vi "Lockin-4461_Multiple Inputs and Outputs_KH_functional_global_waveform_generalized_f.vi"(8 "stop":bool) -> ()   [LabVIEW 2013]
uses:
  <vilib>/Analysis/baseanly.llb/Mean (DBL).vi
  <vilib>/Analysis/2dsp.llb/Decimate (single shot).vi
  <vilib>/Analysis/2dsp.llb/Decimate (single shot, DBL).vi
  DAQ-Lockin-SubVI/Lock-in Globles Multiple Inputs and Outputs used with FGV.vi
  <vilib>/Utility/error.llb/Error Cluster From Error Code.vi
  <vilib>/measure/madcrms.llb/Basic Averaged DC-RMS for 1 Chan.vi
  <vilib>/DAQmx/write.llb/DAQmx Write (Analog 1D Wfm NChan NSamp).vi
  <vilib>/Analysis/NI_AALBase.lvlib
  <vilib>/measure/NI_MAPro.lvlib
  <userlib>/_OpenG.lib/comparison/comparison.llb/Variant Changed__ogtk.vi
panel:
  in  "Boolean":bool
  in  "`":i8(slide) scale=1.0..8.0
  in  "AI Buffer Size":dbl
  in  "order":dbl
  in  "AI Block Size":dbl
  in  "TC (s)":dbl
  in  "Cluster 2":T1
  in  "Enum":enum16{"X and Y", "R and Theta"}(ring)
  in  "Tab Control 3":enum32{"Page 1", "Page 2"}(tab)
  in  "auto controI block size":bool
  in  "zero offset":bool
  in  "measure offset":bool
  in  "reset signal?":bool
  in  "demod = AO?":bool
  in  "all frequencies same?":bool
  in  "simulate?":bool
  in  "Input Signals":i16(slide)=1 scale=1.0..20.0
  out "phase log":dbl[](array[numeric])
  in  "Tab Control 2":T2(tab)=enum."Lock-in Settings"
  in  "AI Configuration":T3(array[cluster])=[{"AI.Coupling"=10050, "AI.Max"=10.0, "AI.Min"=-10.0, "Input physical channels"="PXI1Slot2/ai0:1"}, {"AI.Coupling"=10050, "AI.Max"=10.0, "AI.Min"=-10.0, "Input physical channels"="PXI1Slot3/ai0:1"}, {"AI.Coupling"=10050, "AI.Max"=10.0, "AI.Min"=-10.0, "Input physical channels"="PXI1Slot5/ai0:1"}, {"AI.Coupling"=10050, "AI.Max"=10.0, "AI.Min"=-10.0, "Input physical channels"="PXI1Slot6/ai0:1"}] {"AI.Coupling" items=["AC"=10045, "DC"=10050, "GND"=10066]}
  in  "AO Configuration":T4(array[cluster])=[{"Output physical channels"="PXI1Slot2/ao0:1", "AO. Max"=0.1, "AO.Min"=-0.1}, {"Output physical channels"="PXI1Slot3/ao0:1", "AO. Max"=0.25, "AO.Min"=-0.25}, {"Output physical channels"="PXI1Slot5/ao0:1", "AO. Max"=0.1, "AO.Min"=-0.1}, {"Output physical channels"="PXI1Slot6/ao0:1", "AO. Max"=0.1, "AO.Min"=-0.1}]
  in  "Lockin":T5={"REF f (Hz)"=[13.0, 13.0, 13.0, 13.0, 13.0, 13.0, 13.0, 13.0], "REF phi (deg)"=[0.0, 0.0, 0.0, 0.0, 0.0, 0.0, 0.0, 0.0]} {"REF phi (deg)" format="%#_3g"}
  in  "REF f = AO f?":bool
  in  "Gain":dbl[](array[numeric])=[1.0, 1.0, 1.0, 1.0, 1.0, 1.0, 1.0, 1.0]
  out "elapsed time":dbl=1410.416
  in  "zero offset":bool
  in  "measure offset":bool
  out "AI Rate":dbl=204800.0 format="%.2p"
  out "filter fC (Hz)":dbl=0.3183098861837907
  in  "TC (s)":dbl=0.5
  in  "order":i32=2
  in  "AO":T6={"AO amp (V)"=[0.1, 0.09, 0.08, 0.07, 0.06, 0.05, 0.04, 0.03], "AO DC (V)"=[0.0, 0.0, 0.0, 0.0, 0.0, 0.0, 0.0, 0.0], "AO f (Hz)"=[13.0, 13.0, 13.0, 13.0, 13.0, 13.0, 13.0, 13.0], "AO phi (deg)"=[0.0, 0.0, 0.0, 0.0, 0.0, 0.0, 0.0, 0.0], "function"=[enum."Sine Wave", enum."Sine Wave", enum."Sine Wave", enum."Sine Wave", enum."Sine Wave", enum."Sine Wave", enum."Sine Wave", enum."Sine Wave"]} {"AO DC (V)" format="%#_6p"; "AO amp (V)" format="%#_6p"}
  in  "all  f same?":bool
  in  "simulate?":bool=TRUE
  in  "reset signal":bool
  in  "AI Buffer Size (S)":i32=10
  in  "AI Block Size":i32=15753 format="%.2p"
  in  "milliseconds to wait":u32=1000
  out "sampling info":cluster{"Fs":dbl, "#s":dbl}={"Fs"=204800.0, "#s"=15753.0}
  in  "pre filter fl":dbl=40.0
  in  "prefilter?":bool
  in  "reset REF phi to zero":bool
  in  "autophase?":bool
  in  "auto block size":bool=TRUE
  in  "P":dbl=0.5 format="%.2f"
  in  "I":dbl=0.6 format="%.2f"
  in  "D":dbl=0.019999999999999997 format="%.2f"
  out "Display 2":dbl=-0.01728566342801391 format="%.6p"
  out "Display 1":dbl=0.09985345527594 format="%.6p"
  in  "Display":enum16{"X and Y", "R and Theta"}(ring)=enum."R and Theta"
  out "AO Task":refnum<k21>[](array[refnum])
  out "AI task":refnum<k21>[](array[refnum])
  in  "Tab Control":T7(tab)
  out "Display Y (or Theta) 2":dbl[](graph)
  out "Display X (or R)":waveform(dbl)[](graph)=[{"t0"=timestamp(3507304728.547973 s since 1904-01-01), "dt"=1.0, "Y"=[0.09985345527594]}, {"t0"=timestamp(3507304728.547973 s since 1904-01-01), "dt"=1.0, "Y"=[0.090216464470275]}, {"t0"=timestamp(3507304728.547973 s since 1904-01-01), "dt"=1.0, "Y"=[0.07984767344892373]}, {"t0"=timestamp(3507304728.547973 s since 1904-01-01), "dt"=1.0, "Y"=[0.06948646282319876]}, {"t0"=timestamp(3507304728.547973 s since 1904-01-01), "dt"=1.0, "Y"=[0.0610513314084819]}, {"t0"=timestamp(3507304728.547973 s since 1904-01-01), "dt"=1.0, "Y"=[0.0501207617290639]}, {"t0"=timestamp(3507304728.547973 s since 1904-01-01), "dt"=1.0, "Y"=[0.04039608724889331]}, {"t0"=timestamp(3507304728.547973 s since 1904-01-01), "dt"=1.0, "Y"=[0.029866562813137317]}]
  out "Display Y (or Theta)":waveform(dbl)[](graph)=[{"t0"=timestamp(3507304728.547973 s since 1904-01-01), "dt"=1.0, "Y"=[-0.01728566342801391]}, {"t0"=timestamp(3507304728.547973 s since 1904-01-01), "dt"=1.0, "Y"=[-0.32961665980326604]}, {"t0"=timestamp(3507304728.547973 s since 1904-01-01), "dt"=1.0, "Y"=[-0.26399334892304605]}, {"t0"=timestamp(3507304728.547973 s since 1904-01-01), "dt"=1.0, "Y"=[-0.3359989409283301]}, {"t0"=timestamp(3507304728.547973 s since 1904-01-01), "dt"=1.0, "Y"=[0.18728664235110717]}, {"t0"=timestamp(3507304728.547973 s since 1904-01-01), "dt"=1.0, "Y"=[0.053789543137479]}, {"t0"=timestamp(3507304728.547973 s since 1904-01-01), "dt"=1.0, "Y"=[0.07133775541983144]}, {"t0"=timestamp(3507304728.547973 s since 1904-01-01), "dt"=1.0, "Y"=[-0.34211850150716916]}]
  in  "\"master\" lockin channel":i32
  out "Waveform Graph":waveform(dbl)[](graph)
  in  "decimating factor":i32=1
  out "dt":dbl format="%#_6p"
  in  "decimating factor 2":i32=1
  out "Results (X, Y, R, Theta)":dbl[][](array[numeric])=[[0.09985345073171382, -3.0124962231235766e-05, 0.09985345527594, -0.01728566342801391], [0.09021497158081004, -0.0005190030732351189, 0.090216464470275, -0.32961665980326604], [0.07984682588549666, -0.0003679010969547394, 0.07984767344892373, -0.26399334892304605], [0.0694852680113616, -0.00040748628079075754, 0.06948646282319876, -0.3359989409283301], [0.06105100524667845, 0.0001995623169072153, 0.0610513314084819, 0.18728664235110717], [0.050120739641995225, 4.705359630329193e-05, 0.0501207617290639, 0.053789543137479], [0.04039605593746594, 5.029629532938592e-05, 0.04039608724889331, 0.07133775541983144], [0.02986603038399768, -0.0001783350027455678, 0.029866562813137317, -0.34211850150716916]] format="%#_6p"
  out "offsets":dbl[](array[numeric])
  out "phase out":dbl[](array[numeric])=[269.2599609379251, 269.2406250004251, 269.2212890629251, 269.2019531254251, 269.18261718792513, 269.16328125042514, 269.14394531292515, 269.12460937542517]
  in  "Phase&Tc":T8(array[cluster])=[{"Phase"=0.0, "Time constant"=0.5, "Set Tc"=FALSE, "Autophase"=FALSE, "Order"=0.0}, {"Phase"=0.0, "Time constant"=0.5, "Set Tc"=FALSE, "Autophase"=FALSE, "Order"=0.0}, {"Phase"=0.0, "Time constant"=0.5, "Set Tc"=FALSE, "Autophase"=FALSE, "Order"=0.0}, {"Phase"=0.0, "Time constant"=0.5, "Set Tc"=FALSE, "Autophase"=FALSE, "Order"=0.0}, {"Phase"=0.0, "Time constant"=0.5, "Set Tc"=FALSE, "Autophase"=FALSE, "Order"=0.0}, {"Phase"=0.0, "Time constant"=0.5, "Set Tc"=FALSE, "Autophase"=FALSE, "Order"=0.0}, {"Phase"=0.0, "Time constant"=0.5, "Set Tc"=FALSE, "Autophase"=FALSE, "Order"=0.0}, {"Phase"=0.0, "Time constant"=0.5, "Set Tc"=FALSE, "Autophase"=FALSE, "Order"=0.0}] {"Phase" min=0.0 max=360.0 scale=0.0..360.0}
  in  "sample clock multiple (x*f)":i32=1000
  # "SIMPLIFY THIS !!!!!!!!!!!!!!!!!!!!!!!!!!!!!!!!!!!!!!!!!!!!!!!!!!!!!!!!!!"
  # "Real time Adjustable Values"
  # "WAVEFORM 2"
  # "Configurations"
  # "should this be x multiple\nof the frequency?"
  # "Features:\n1, Any number of input and output channels\n2, Each AO outputs an DC+AC signal, DC for sample biasing and AC for OSC. These values can be adjusted in real time.\n3, Synchronous filtering\n\nInstructions:\n1, Array index of AI configuration and AO configuration refers to task.\n2, Array index in Amplifier Settings, Phase$&Tc control , and gains correlates to channel number.\n3, Each 4461 board can have 2 lock-in channels. Syntax for 2 channles, e.g. PXI1Slot2/ai0:1. If you want to use just one, then PXI1Slot2/ai0.\n4, Parameters (especially DC value for sample biasing) can be remotely controlled by clicking \"local\"and \"remote\" button. In real experiments, put golable values (can be found in Lock-in globles.vi) in your VI to control the lock-in and read out.\n5, choose OSC frequencies to be multiple of \nAI Rate/AI Block SIze to have best performance.\n\n-Guanglei 06/23/2011\n\nUpdate:\n1. Allows any number of lockin amplifiers and AO tasks.\n2. Delete the channels from any AI/AO Configuration elements you do not want to use.\n3. Rows (first index) of the OSC Configuration correspond to different AO tasks, while columns (second index) correspond to AO channels in that task. All channels in a given element of the AO Configuration array will go into a single task.\n4. The same number of output channels must go in each AO task.\n5. Make sure a Phase&Tc element and an Amplifier Settings element is set for each AI channel.\n-Joe 12/3/2013"
  # "signal\n*sine\n*cosine\n*2\n*2\nLP filter\nLP filter"
  # "auto decimate so total # points is certain value? (O 1000?)"
  # "hide stuff here in this tab"
  # "multiple of frequency??"
  # "this is \"time constant\""
  # "The top array index selects which card you are setting the outputs for,and the second index selects which output chanel on that card.\n\nFor Phase&Tc, you must have an array element initialized for each input signal."
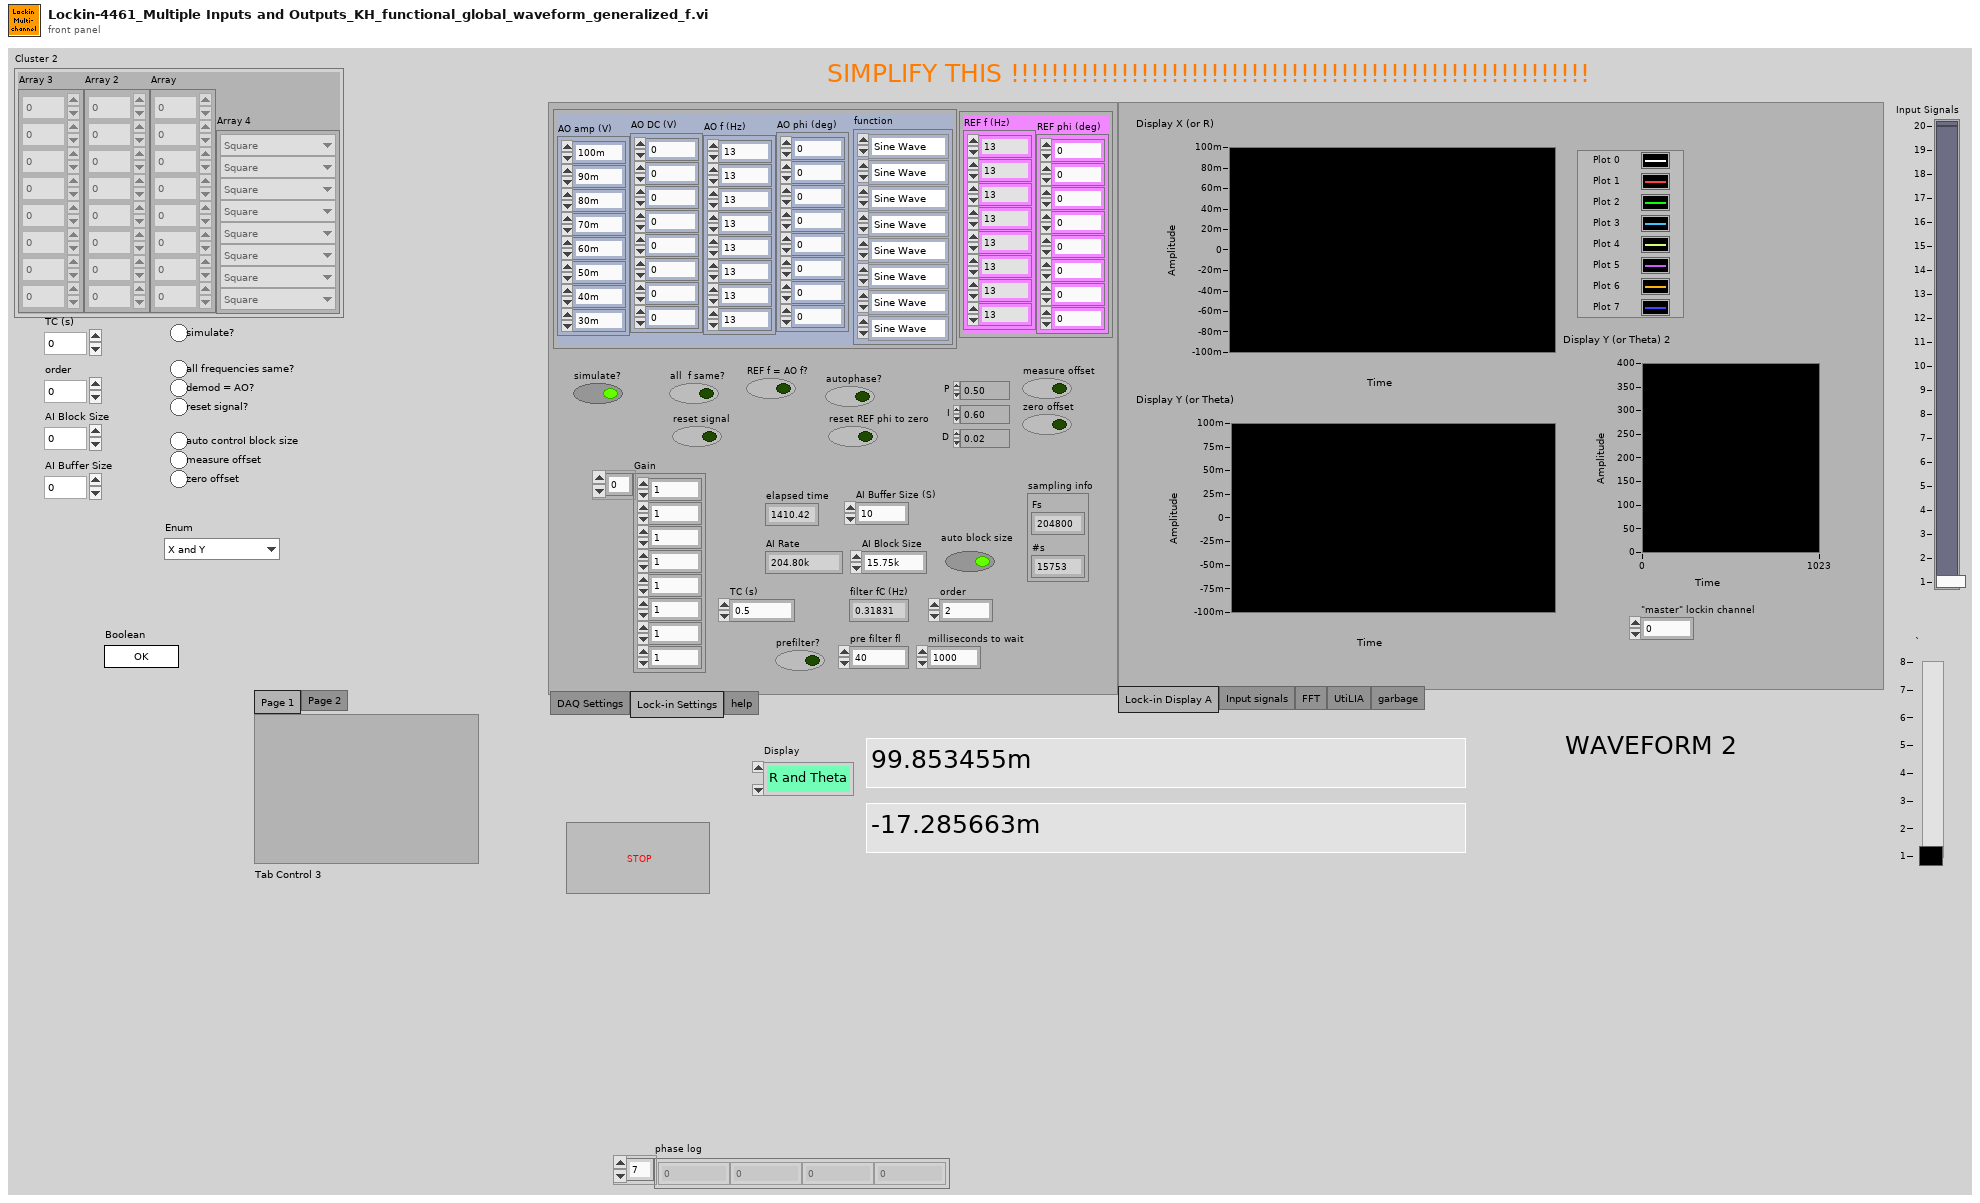
[diagram p1: front panel]
types:
  T1 = cluster{"Array":dbl[], "Array 2":dbl[], "Array 3":dbl[], "Array 4":enum16{"Square\n", "Sine", "Triangle"}[]}
  T2 = enum32{"DAQ Settings", "Lock-in Settings", "help"}
  T3 = cluster{"AI.Coupling":i32, "AI.Max":dbl, "AI.Min":dbl, "Input physical channels":tag}[]
  T4 = cluster{"Output physical channels":tag, "AO. Max":dbl, "AO.Min":dbl}[]
  T5 = cluster{"REF f (Hz)":dbl[], "REF phi (deg)":dbl[]}
  T6 = cluster{"AO amp (V)":dbl[], "AO DC (V)":dbl[], "AO f (Hz)":dbl[], "AO phi (deg)":dbl[], "function":enum16{"Sine Wave", "Triangle Wave", "Square Wave", "Sawtooth Wave"}[]}
  T7 = enum32{"Lock-in Display A", "Input signals", "FFT", "UtiLIA", "garbage"}
  T8 = cluster{"Phase":dbl, "Time constant":dbl, "Set Tc":bool, "Autophase":bool, "Order":dbl}[]
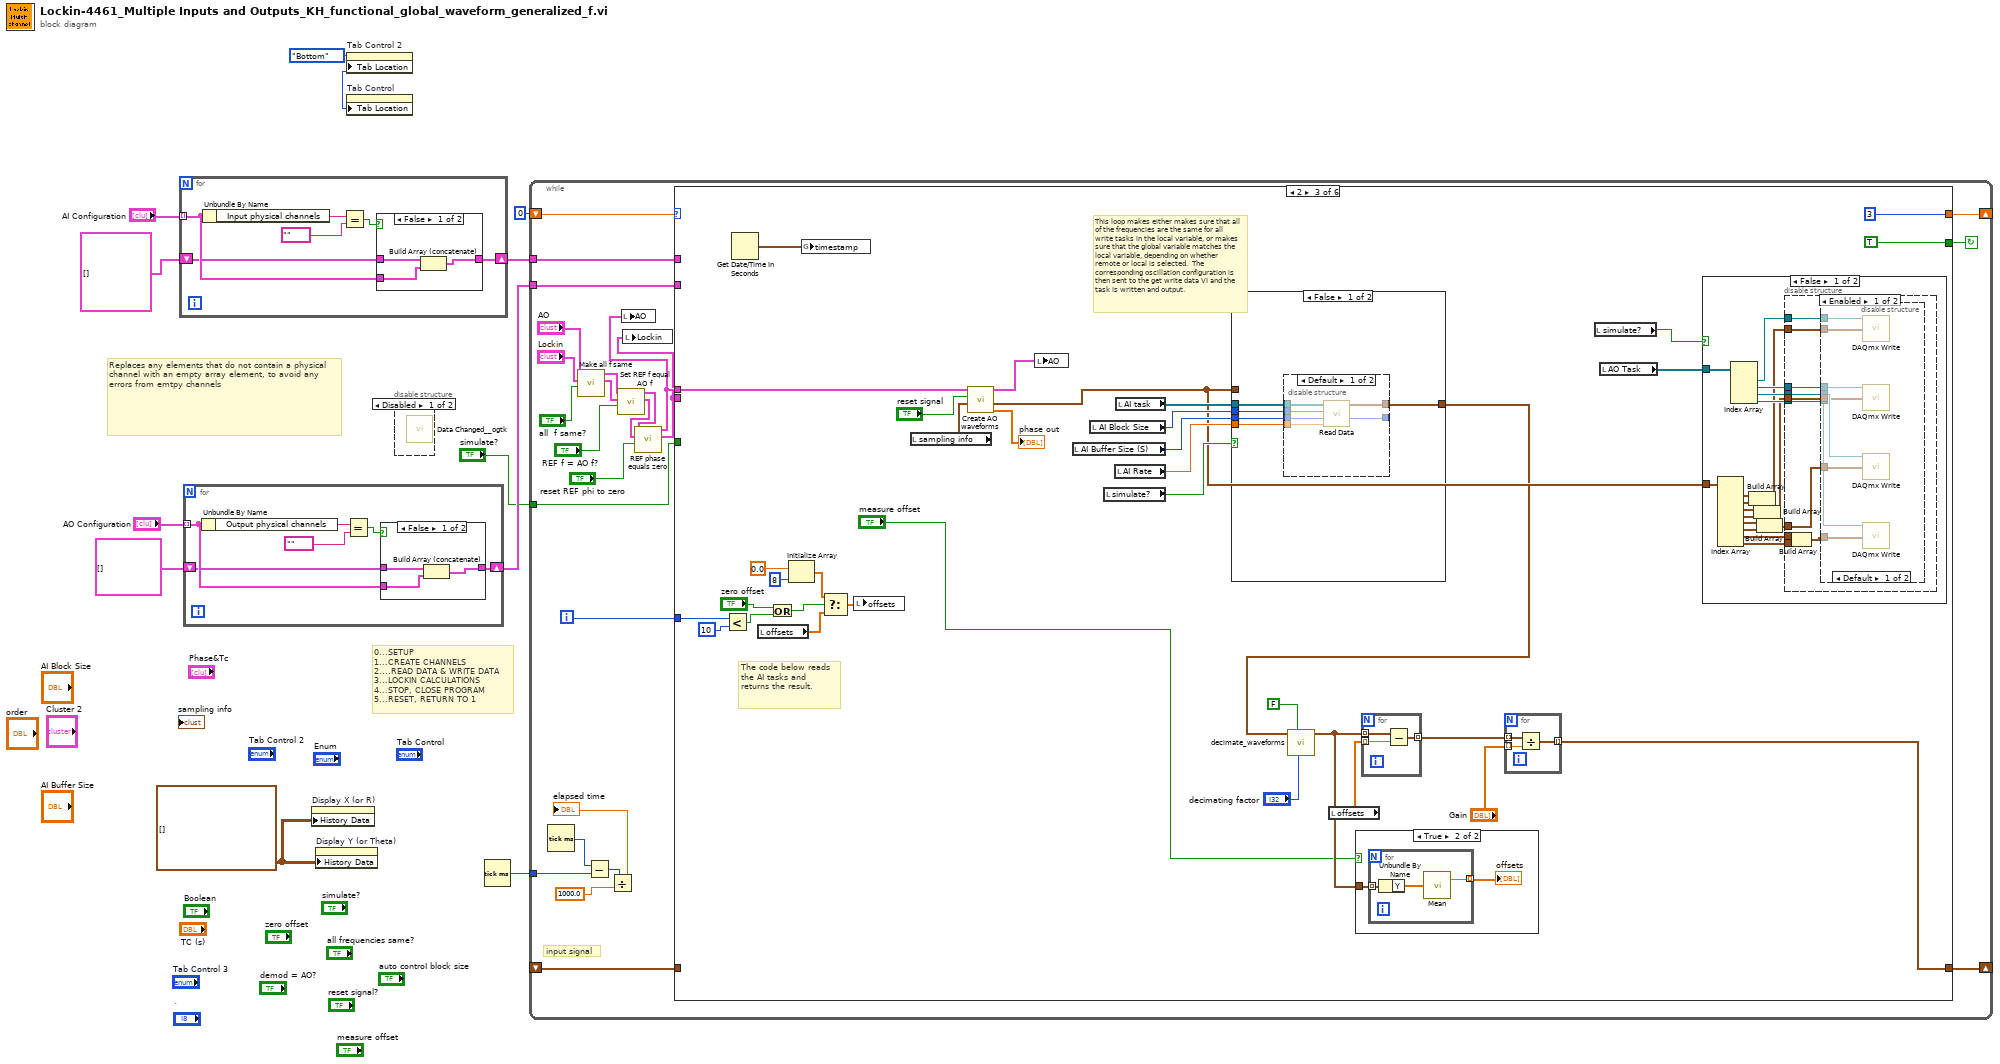
[diagram p0: block diagram]
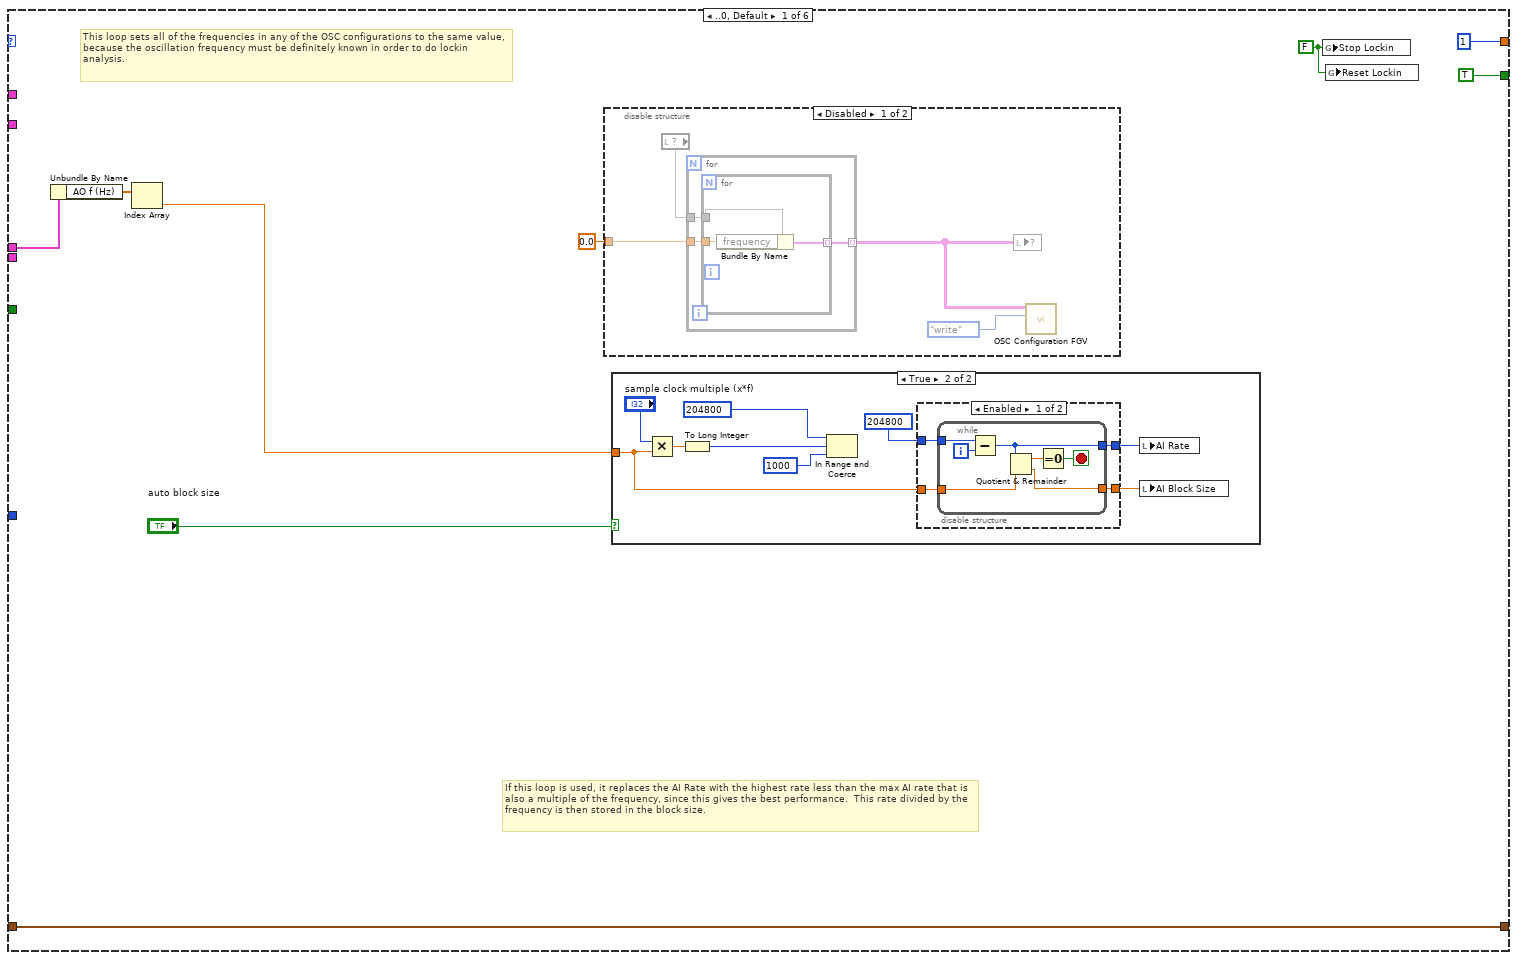
[diagram p5: hidden frame]
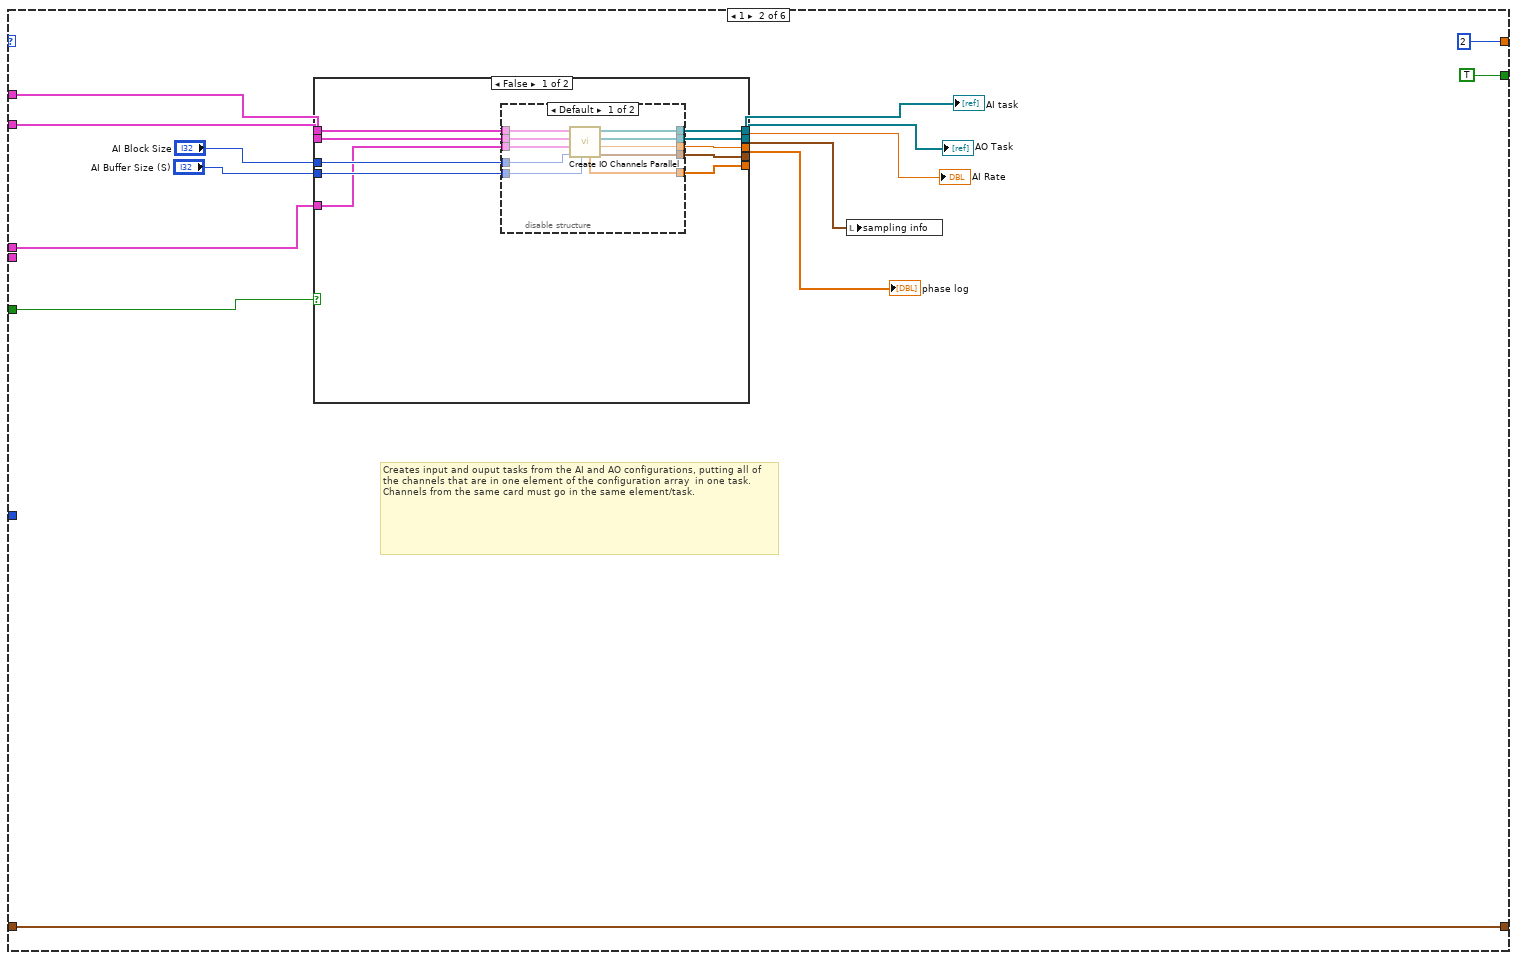
[diagram p9: hidden frame]
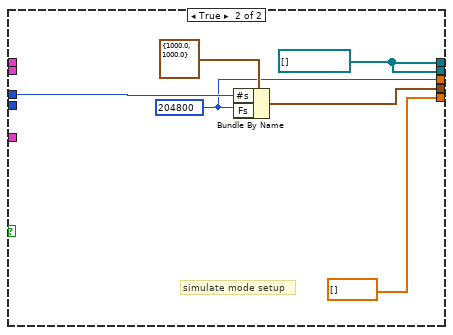
[diagram p11: hidden frame]
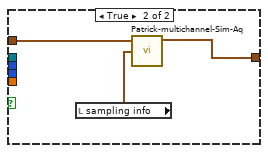
[diagram p16: hidden frame]
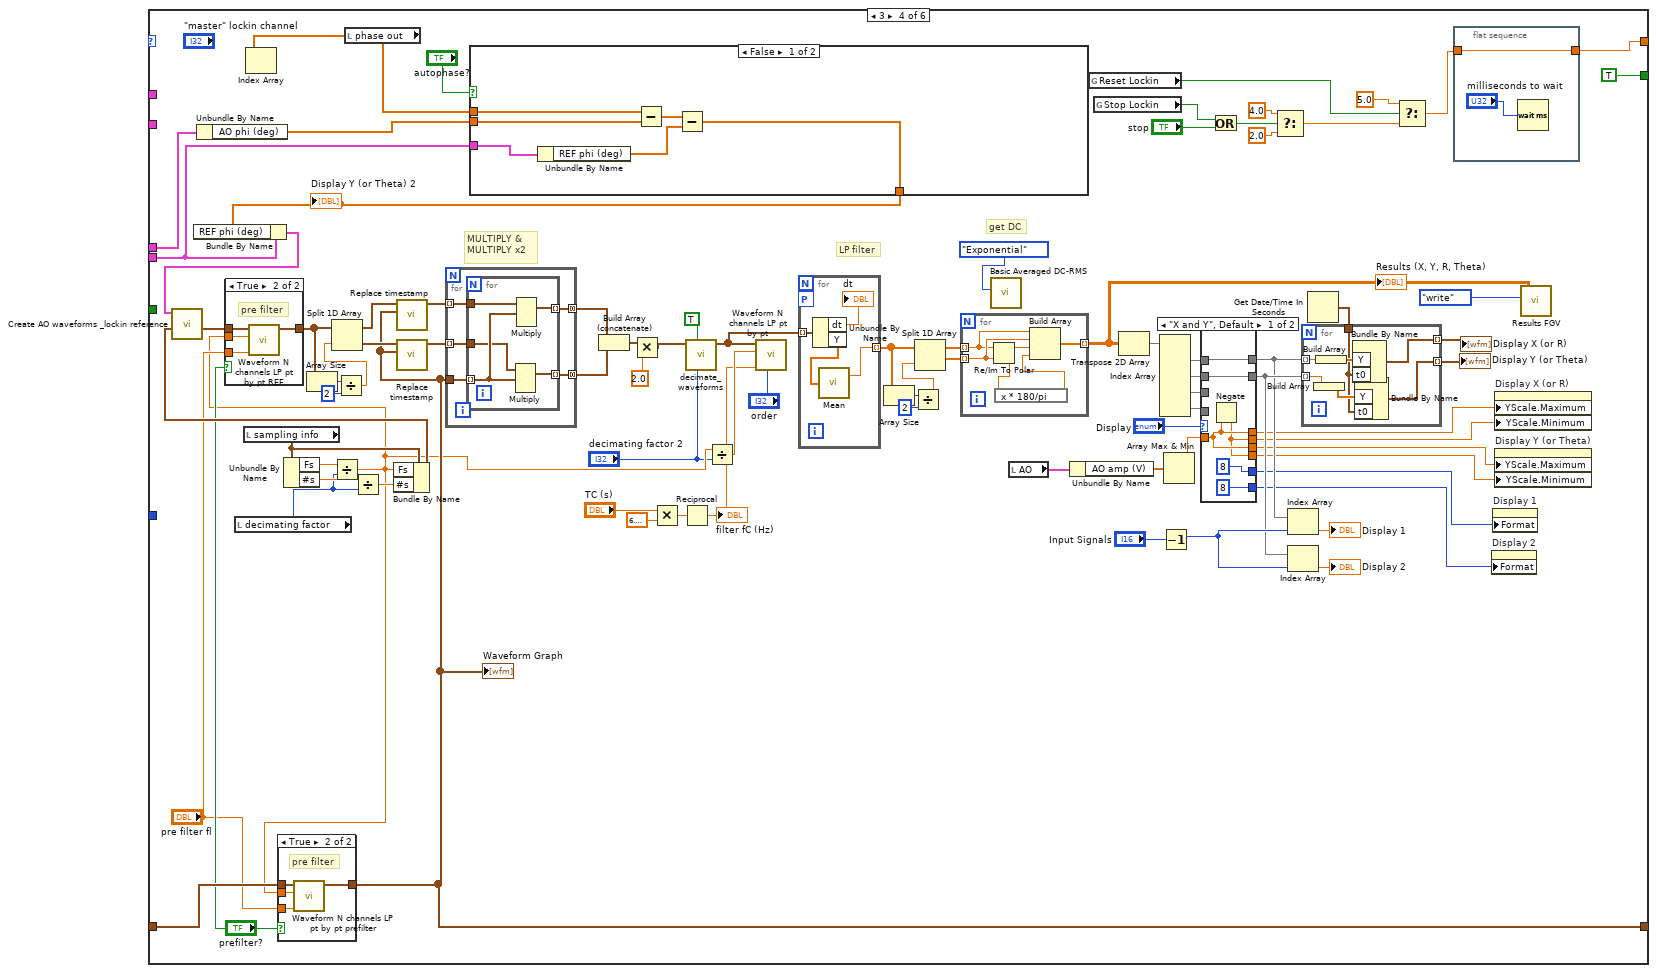
[diagram p18: hidden frame]
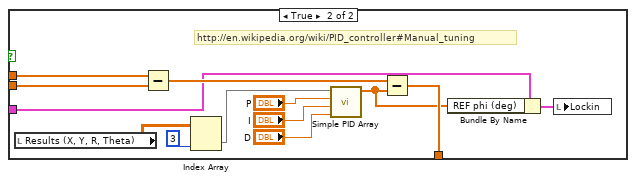
[diagram p20: hidden frame]
diagram:
  w2 = waveform(dbl)[][] [] ("History Data")
  w6 = enum32{"Top", "Bottom", "Left", "Right"}."Bottom" ("Tab Location")
  # "0...SETUP\n1...CREATE CHANNELS\n2....READ DATA & WRITE DATA\n3...LOCKIN CALCULATIONS\n4...STOP, CLOSE PROGRAM\n5...RESET, RETURN TO 1"
  # "Replaces any elements that do not contain a physical channel with an empty array element, to avoid any errors from emtpy channels"
  n1 = for {
    tunnel: "AI Configuration" -> [w14] mode=indexing
    shift-right: [w12] -> w11
    shift-left: T3 [] ("AI Configuration") -> [w13]
    n2 = Unbundle By Name(w14) -> ("Input physical channels"=w16:tag)
    n3 = Equal?(x=w16, y=tag "" ("Empty physical channels")) -> (x = y?=w17:bool)
    n4 = case shown="False" w17 {
      tunnel: w14 -> [w19 _]
      tunnel: w13 -> [w20 w21]
      tunnel: [w18 w21] -> w12
      frame False {
        n5 = Build Array (concatenate)(w20, w19) -> (w18:T3)
      }
      frame True {
      }
    }
  }
  n6 = for {
    tunnel: "AO Configuration" -> [w24] mode=indexing
    shift-right: [w22] -> w4
    shift-left: T4 [] ("AO Configuration 2") -> [w23]
    n7 = Unbundle By Name(w24) -> ("Output physical channels"=w26:tag)
    n8 = Equal?(x=w26, y=tag "" ("Empty physical channels")) -> (x = y?=w27:bool)
    n9 = case shown="False" w27 {
      tunnel: w24 -> [w29 _]
      tunnel: w23 -> [w30 w31]
      tunnel: [w28 w31] -> w22
      frame False {
        n10 = Build Array (concatenate)(w30, w29) -> (w28:T4)
      }
      frame True {
      }
    }
  }
  n11 = property on="Display X (or R)" class="WaveformChart (strict)"("History Data"=w2) -> ()  [unwired: 2 in, 2 out]
  n12 = property on="Display Y (or Theta)" class="WaveformChart (strict)"("History Data"=w2) -> ()  [unwired: 2 in, 2 out]
  n13 = property on="Tab Control 2" class="TabCtl (strict)"("Tab Location"=w6) -> ()  [unwired: 2 in, 2 out]
  n14 = property on="Tab Control" class="TabCtl (strict)"("Tab Location"=w6) -> ()  [unwired: 2 in, 2 out]
  n15 = disable-structure shown="Disabled" {
    frame Disabled {
      n16 = call-poly <userlib>:"Data Changed__ogtk.vi"() -> ()  [unwired: 1 in, 1 out]
    }
    frame Enabled {
    }
  }
  n17 = Tick Count (ms)() -> (millisecond timer value=w3:u32)
  n18 = while {
    shift-right: [w56] -> _
    shift-left: 0 -> [w55]
    tunnel: w11 -> [w54]
    tunnel: w4 -> [w53]
    shift-right: [w52] -> _
    shift-left: _ -> [w51]
    tunnel: w3 -> [w50]
    tunnel: "simulate?" -> [w32]
    i -> [w47]
    stop <- w48 continue-if-true
    # "input signal"
    n19 = Tick Count (ms)() -> (millisecond timer value=w46:u32)
    n20 = call "Make all f same.vi"("all  frequencies same?"="all  f same?", "Lockin"="Lockin", "AO"="AO") -> ("Lockin 2"=w39:T5, "AO 2"=w40:T6)  [unwired: 7 in]
    n21 = Subtract(x=w46, y=w50) -> (x-y=w49:u32)
    n22 = Divide(x=w49, y=1000.0) -> (x/y=→"elapsed time":dbl)
    n23 = call "Set REF f equal AO f.vi"("REE = AO?"="REF f = AO f?", "Lockin"=w39, "AO"=w40) -> ("Lockin 2"=w37:T5, "AO 2"=w38:T6)  [unwired: 7 in]
    n24 = call "REF phase equals zero.vi"("reset REF phi to zero"="reset REF phi to zero", "Lockin"=w37, "AO"=w38) -> ("Lockin 2"=w33:T5, "AO 2"=w34:T6)  [unwired: 7 in]
    n25 = local write "AO"(w34) -> ()
    n26 = local write "Lockin"(w33) -> ()
    n27 = case shown="2" w55 {
      selector: w55 -> [_ _ _ _ w392 _]
      tunnel: [1 2 3 w288 w392 0.0 ("f")] -> w56
      tunnel: w54 -> [_ w109 _ _ _ _]
      tunnel: [TRUE TRUE TRUE TRUE FALSE TRUE] -> w48
      tunnel: w53 -> [_ w108 _ _ _ _]
      tunnel: [w61 w105 w147 w258 w391 w421] -> w52
      tunnel: w51 -> [w61 w105 _ w280 w391 w421]
      tunnel: w47 -> [_ _ w165 _ _ _]
      tunnel: w32 -> [_ w102 _ _ _ _]
      tunnel: w34 -> [w59 w98 w142 w252 _ _]
      tunnel: w33 -> [_ _ _ w257 _ _]
      frame ..0, Default {
        w64 = FALSE ("Stop Lockin")
        # "If this loop is used, it replaces the AI Rate with the highest rate less than the max AI rate that is also a multiple of the frequency, since this gives the best performance.  This rate divided by the frequency is then stored in the block size."
        # "This loop sets all of the frequencies in any of the OSC configurations to the same value, because the oscillation frequency must be definitely known in order to do lockin analysis."
        n28 = Unbundle By Name(w59) -> ("AO f (Hz)"=w58:dbl[])
        n29 = Index Array(array=w58) -> (element=w57:dbl)  [unwired: 1 in]
        n30 = disable-structure shown="Disabled" {
          disable-tunnel: 0.0 -> [w66 _]
          frame Disabled {
            n31 = local read item#-1() -> (w69)
            n32 = for {
              tunnel: w69 -> [w72]
              tunnel: [w71] -> w68 mode=indexing
              tunnel: w66 -> [w70]
              n33 = for {
                tunnel: w72 -> [w75]
                tunnel: [w74] -> w71 mode=indexing
                tunnel: w70 -> [w73]
                n34 = Bundle By Name(cluster=w75, "frequency"=w73) -> (w74:cluster{})
              }
            }
            n35 = local write item#-1(w68) -> ()
            n36 = call "OSC Configuration FGV.vi"("Function"=enum16{"write", "read"}."write", "OSC Configuration"=w68) -> ()  [unwired: 4 in, 2 out]
          }
          frame Enabled {
          }
        }
        n37 = case shown="True" "auto block size" {
          tunnel: w57 -> [_ w76]
          frame False {
          }
          frame True {
            n38 = Multiply(x="sample clock multiple (x*f)", y=w76) -> (x*y=w82:dbl)
            n39 = To Long Integer(number=w82) -> (32bit integer=w80:i32)
            n40 = In Range and Coerce(upper limit=204800, x=w80, lower limit=1000) -> ()  [unwired: 2 out]
            n41 = disable-structure shown="Enabled" {
              disable-tunnel: [w88 w96] -> w84
              disable-tunnel: [w87 w97] -> w83
              disable-tunnel: 204800 ("max ai rate") -> [w86 w97]
              disable-tunnel: w76 -> [w85 w96]
              frame Enabled {
                n42 = while {
                  tunnel: w86 -> [w95]
                  tunnel: [w93] -> w88
                  tunnel: [w91] -> w87
                  tunnel: w85 -> [w92]
                  i -> [w94]
                  stop <- w89 stop-if-true
                  n43 = Subtract(x=w95, y=w94) -> (x-y=w91:i32)
                  n44 = Quotient & Remainder(x=w91, y=w92) -> (x-y*floor(x/y)=w90:dbl, floor(x/y)=w93:dbl)
                  n45 = Equal To 0?(x=w90) -> (x = 0?=w89:bool)
                }
              }
              frame Disabled {
              }
            }
            n46 = local write "AI Rate"(w83) -> ()
            n47 = local write "AI Block Size"(w84) -> ()
          }
        }
        n48 = global write "Lock-in Globles Multiple Inputs and Outputs used with FGV.vi" "Stop Lockin"(w64) -> ()
        n49 = global write "Lock-in Globles Multiple Inputs and Outputs used with FGV.vi" "Reset Lockin"(w64) -> ()
      }
      frame 1 {
        # "Creates input and ouput tasks from the AI and AO configurations, putting all of the channels that are in one element of the configuration array  in one task.  Channels from the same card must go in the same element/task."
        n50 = case shown="False" w102 {
          tunnel: w109 -> [w121 _]
          tunnel: w108 -> [w120 _]
          tunnel: [w119 w137] -> w107
          tunnel: [w118 w132] -> w106
          tunnel: "AI Block Size" -> [w117 w136]
          tunnel: [w116 w135] -> w101
          tunnel: [w115 w137] -> w104
          tunnel: "AI Buffer Size (S)" -> [w114 _]
          tunnel: [w113 dbl[] [] ("phase log")] -> w103
          tunnel: w98 -> [w112 _]
          frame False {
            n51 = disable-structure shown="Default" {
              disable-tunnel: w121 -> [w131 _]
              disable-tunnel: w120 -> [w130 _]
              disable-tunnel: [w129 _] -> w119
              disable-tunnel: [w128 _] -> w118
              disable-tunnel: w117 -> [w123 _]
              disable-tunnel: [w127 _] -> w116
              disable-tunnel: [w126 _] -> w115
              disable-tunnel: w114 -> [w125 _]
              disable-tunnel: [w124 _] -> w113
              disable-tunnel: w112 -> [w122 _]
              frame condition #0 {
                n52 = call "Create IO Channels Parallel.vi"("AI Buffer Size (s)"=w125, "AI Block Size"=w123, "AO"=w122, "AO Configuration"=w130, "AI Configuration"=w131) -> ("sampling info"=w127:cluster{"Fs":dbl, "#s":dbl}, "AI Rate"=w128:dbl, "AO Task"=w126:refnum<k21>[], "AI task"=w129:refnum<k21>[], "phase log"=w124:dbl[])  [unwired: 1 in, 1 out]
              }
              frame condition #1 (active) {
              }
            }
          }
          frame True {
            w132 = 204800 ("index (row)")
            w137 = refnum<k21>[] [] ("AI task")
            # "simulate mode setup"
            n53 = Bundle By Name(cluster=cluster{"Fs":dbl, "#s":dbl} {"Fs"=1000.0, "#s"=1000.0} ("sampling info"), "#s"=w136, "Fs"=w132) -> (w135:cluster{"Fs":dbl, "#s":dbl})
          }
        }
        "AO Task" <- w104
        "AI Rate" <- w106
        "AI task" <- w107
        "phase log" <- w103
        n54 = local write "sampling info"(w101) -> ()
      }
      frame 2 {
        # "The code below reads the AI tasks and returns the result."
        # "This loop makes either makes sure that all of the frequencies are the same for all write tasks in the local variable, or makes sure that the global variable matches the local variable, depending on whether remote or local is selected.  The corresponding oscillation configuration is then sent to the get write data VI and the task is written and output."
        n55 = Less?(x=w165, y=10) -> (x < y?=w158:bool)
        n56 = Get Date/Time In Seconds() -> (seconds since 1Jan1904=w170:timestamp)
        n57 = local read "offsets"() -> (w164:dbl[])
        n58 = Or(x="zero offset", y=w158) -> (x .or. y?=w157:bool)
        n59 = Initialize Array(0.0, 8 ("dimension size")) -> (w161:dbl[])
        n60 = global write "Lock-in Globles Multiple Inputs and Outputs used with FGV.vi" "timestamp"(w170) -> ()
        n61 = Select(t=w161, s=w157, f=w164) -> (s? t:f=w163:dbl[])
        n62 = local write "offsets"(w163) -> ()
        n63 = local read "sampling info"() -> (w144:cluster{"Fs":dbl, "#s":dbl})
        n64 = call "Create AO waveforms.vi"("sampling info"=w144, "reset signal"="reset signal", "AO"=w142) -> ("phase out"=→"phase out":dbl[], "AO Array"=w139:waveform(dbl)[], "AO 2"=w145:T6)  [unwired: 6 in]
        n65 = local write "AO"(w145) -> ()
        n66 = local read "AI Buffer Size (S)"() -> (w168:i32)
        n67 = local read "AI Block Size"() -> (w169:i32)
        n68 = local read "simulate?"() -> (w146:bool)
        n69 = local read "AI Rate"() -> (w167:dbl)
        n70 = local read "AI task"() -> (w148:refnum<k21>[])
        n71 = case shown="False" w146 {
          tunnel: w148 -> [w212 _]
          tunnel: w169 -> [w211 _]
          tunnel: w168 -> [w210 _]
          tunnel: w167 -> [w209 _]
          tunnel: [w208 w221] -> w138
          tunnel: w139 -> [_ w219]
          frame False {
            n72 = disable-structure shown="Default" {
              disable-tunnel: w212 -> [w218 _]
              disable-tunnel: w211 -> [w217 _]
              disable-tunnel: w210 -> [w216 _]
              disable-tunnel: w209 -> [w215 _]
              disable-tunnel: [w214 _] -> _
              disable-tunnel: [w213 _] -> w208
              frame condition #0 {
                n73 = call "Read Data.vi"("AI Rate"=w215, "AI Buffer Size (s)"=w216, "AI Block Size"=w217, "AI task"=w218) -> ("Backlog"=w214:u8, "Input Signals"=w213:waveform(dbl)[])  [unwired: 5 in, 1 out]
              }
              frame condition #1 (active) {
              }
            }
          }
          frame True {
            n74 = local read "sampling info"() -> (w220:cluster{"Fs":dbl, "#s":dbl})
            n75 = call "Patrick-multichannel-Sim-Aq.vi"("data"=w219, "sampling info"=w220) -> ("Data"=w221:waveform(dbl)[])  [unwired: 5 in]
          }
        }
        n76 = call "decimate_waveforms.vi"("decimating factor"="decimating factor", "averaging"=FALSE, "Input Signal"=w138) -> ("Decimated Waveforms"=w152:waveform(dbl)[])  [unwired: 7 in, 1 out]
        n77 = local read "offsets"() -> (w156:dbl[])
        n78 = case shown="True" "measure offset" {
          tunnel: w152 -> [_ w222]
          frame False {
          }
          frame True {
            n79 = for {
              tunnel: [w226] -> w223 mode=indexing
              tunnel: w222 -> [w225] mode=indexing
              n80 = Unbundle By Name(w225) -> ("Y"=w224:dbl[])
              n81 = call-poly <vilib>:"Mean.vi"("X"=w224) -> ("mean"=w226:dbl)  [unwired: 1 out]
            }
            "offsets" <- w223
          }
        }
        n82 = for {
          tunnel: w152 -> [w229] mode=indexing
          tunnel: [w228] -> w151 mode=indexing
          tunnel: w156 -> [w227] mode=indexing
          n83 = Subtract(x=w229, y=w227) -> (x-y=w228:waveform(dbl))
        }
        n84 = for {
          tunnel: w151 -> [w232] mode=indexing
          tunnel: [w231] -> w147 mode=indexing
          tunnel: "Gain" -> [w230] mode=indexing
          n85 = Divide(x=w232, y=w230) -> (x/y=w231:waveform(dbl))
        }
        n86 = local read "simulate?"() -> (w140:bool)
        n87 = local read "AO Task"() -> (w149:refnum<k21>[])
        n88 = case shown="False" w140 {
          tunnel: w149 -> [w189 _]
          tunnel: w139 -> [w184 _]
          frame False {
            n89 = Index Array(array=w184) -> (element #1=w183:waveform(dbl), element #2=w182:waveform(dbl), element #3=w181:waveform(dbl), element #4=w180:waveform(dbl), element #5=w179:waveform(dbl), element #6=w178:waveform(dbl), element #7=w177:waveform(dbl), element #8=w176:waveform(dbl))  [unwired: 8 in]
            n90 = Index Array(array=w189) -> (element #1=w188:refnum<k21>, element #2=w187:refnum<k21>, element #3=w186:refnum<k21>, element #4=w185:refnum<k21>)  [unwired: 4 in]
            n91 = Build Array(w183, w182) -> (w175:waveform(dbl)[])
            n92 = Build Array(w181, w180) -> (w174:waveform(dbl)[])
            n93 = Build Array(w179, w178) -> (w173:waveform(dbl)[])
            n94 = disable-structure shown="Enabled" {
              disable-tunnel: w188 -> [w199 _]
              disable-tunnel: w187 -> [w198 _]
              disable-tunnel: w186 -> [w197 _]
              disable-tunnel: w185 -> [w196 _]
              disable-tunnel: w177 -> [w195 _]
              disable-tunnel: w176 -> [w194 _]
              disable-tunnel: w175 -> [w193 _]
              disable-tunnel: w174 -> [w192 _]
              disable-tunnel: w173 -> [w191 _]
              frame Enabled {
                n95 = Build Array(w195, w194) -> (w190:waveform(dbl)[])
                n96 = disable-structure shown="Default" {
                  disable-tunnel: w199 -> [w207 _]
                  disable-tunnel: w198 -> [w206 _]
                  disable-tunnel: w197 -> [w205 _]
                  disable-tunnel: w196 -> [w204 _]
                  disable-tunnel: w193 -> [w203 _]
                  disable-tunnel: w192 -> [w202 _]
                  disable-tunnel: w191 -> [w201 _]
                  disable-tunnel: w190 -> [w200 _]
                  frame condition #0 {
                    n97 = call-poly <vilib>:"DAQmx Write.vi"("task/channels in"=w207, "data"=w203) -> ()  [unwired: 11 in, 3 out]
                    n98 = call-poly <vilib>:"DAQmx Write.vi"("task/channels in"=w206, "data"=w202) -> ()  [unwired: 11 in, 3 out]
                    n99 = call-poly <vilib>:"DAQmx Write.vi"("task/channels in"=w205, "data"=w201) -> ()  [unwired: 11 in, 3 out]
                    n100 = call-poly <vilib>:"DAQmx Write.vi"("task/channels in"=w204, "data"=w200) -> ()  [unwired: 11 in, 3 out]
                  }
                  frame condition #1 (active) {
                  }
                }
              }
              frame Disabled {
              }
            }
          }
          frame True {
          }
        }
      }
      frame 3 {
        # "get DC"
        # "LP filter"
        # "MULTIPLY &\nMULTIPLY x2"
        n101 = Unbundle By Name(w252) -> ("AO phi (deg)"=w251:dbl[])
        n102 = local read "decimating factor"() -> (w246:i32)
        n103 = local read "sampling info"() -> (w245:cluster{"Fs":dbl, "#s":dbl})
        n104 = Unbundle By Name(w245) -> ("Fs"=w306:dbl, "#s"=w291:dbl)
        n105 = Divide(x=w306, y=w246) -> (x/y=w244:dbl)
        n106 = case shown="True" "prefilter?" {
          tunnel: w280 -> [w356 w360]
          tunnel: w244 -> [_ w359]
          tunnel: "pre filter fl" -> [_ w358]
          tunnel: [w356 w357] -> w258
          frame False {
          }
          frame True {
            # "pre filter"
            n107 = call "Waveform N channels LP pt by pt prefilter.vi"("fl"=w358, "fs"=w359, "Array in"=w360) -> ("Array out"=w357:waveform(dbl)[])  [unwired: 8 in]
          }
        }
        "Waveform Graph" <- w258
        n108 = local read "phase out"() -> (w237:dbl[])
        n109 = Index Array(array=w237) -> ()  [unwired: 1 in, 1 out]
        n110 = Divide(x=w291, y=w246) -> (x/y=w290:dbl)
        n111 = Bundle By Name(cluster=w245, "Fs"=w244, "#s"=w290) -> (w289:cluster{"Fs":dbl, "#s":dbl})
        n112 = case shown="False" "autophase?" {
          tunnel: [w341 w354] -> w253
          tunnel: w257 -> [w340 w344]
          tunnel: w251 -> [w338 w345]
          tunnel: w237 -> [w337 w343]
          frame False {
            n113 = Unbundle By Name(w340) -> ("REF phi (deg)"=w339:dbl[])
            n114 = Subtract(x=w337, y=w338) -> (x-y=w342:dbl[])
            n115 = Subtract(x=w342, y=w339) -> (x-y=w341:dbl[])
          }
          frame True {
            # "http://en.wikipedia.org/wiki/PID_controller#Manual_tuning"
            n116 = local read "Results (X, Y, R, Theta)"() -> (w352:dbl[][])
            n117 = Subtract(x=w343, y=w345) -> (x-y=w355:dbl[])
            n118 = Index Array(array=w352, index (col)=3 ("index (row)")) -> (element=w351:dbl[])  [unwired: 1 in]
            n119 = call "Simple PID Array.vi"("D"="D", "I"="I", "P"="P", "process variable"=w351) -> ("output value"=w347:dbl[])  [unwired: 7 in]
            n120 = Subtract(x=w355, y=w347) -> (x-y=w354:dbl[])
            n121 = Bundle By Name(cluster=w344, "REF phi (deg)"=w347) -> (w346:T5)
            n122 = local write "Lockin"(w346) -> ()
          }
        }
        "Display Y (or Theta) 2" <- w253
        n123 = Bundle By Name(cluster=w257, "REF phi (deg)"=w253) -> (w256:T5)
        n124 = call "Create AO waveforms _lockin reference.vi"("sampling info"=w289, "Lockin"=w256) -> ("AO Array"=w261:waveform(dbl)[])  [unwired: 7 in, 2 out]
        n125 = case shown="True" "prefilter?" {
          tunnel: w261 -> [w332 w336]
          tunnel: [w332 w335] -> w250
          tunnel: "pre filter fl" -> [_ w334]
          tunnel: w244 -> [_ w333]
          frame False {
          }
          frame True {
            # "pre filter"
            n126 = call "Waveform N channels LP pt by pt REF.vi"("fl"=w334, "fs"=w333, "Array in"=w336) -> ("Array out"=w335:waveform(dbl)[])  [unwired: 8 in]
          }
        }
        n127 = Array Size(array=w250) -> (size(s)=w249:i32)
        n128 = Divide(x=w249, y=2) -> (x/y=w247:dbl)
        n129 = Split 1D Array(array=w250, index=w247) -> (first subarray=w283:waveform(dbl)[], second subarray=w282:waveform(dbl)[])
        n130 = call "Replace timestamp.vi"("Array in"=w258, "Array 2"=w283) -> ("Array"=w262:waveform(dbl)[])  [unwired: 9 in]
        n131 = call "Replace timestamp.vi"("Array in"=w258, "Array 2"=w282) -> ("Array"=w281:waveform(dbl)[])  [unwired: 9 in]
        n132 = for {
          tunnel: [w322] -> w296 mode=concatenating
          tunnel: [w321] -> w295 mode=concatenating
          tunnel: w281 -> [w320] mode=indexing
          tunnel: w262 -> [w319] mode=indexing
          tunnel: w258 -> [w318]
          n133 = for {
            tunnel: [w327] -> w321 mode=indexing
            tunnel: w320 -> [w323]
            tunnel: w318 -> [w325] mode=indexing
            tunnel: w319 -> [w324]
            tunnel: [w326] -> w322 mode=indexing
            n134 = Multiply(1:w325, 2:w323) -> (0:w327:waveform(dbl))  [unwired: 1 in, 1 out]
            n135 = Multiply(1:w325, 2:w324) -> (0:w326:waveform(dbl))  [unwired: 1 in, 1 out]
          }
        }
        n136 = Build Array (concatenate)(w296, w295) -> (w294:waveform(dbl)[])
        n137 = Multiply(x=w294, y=2.0) -> (x*y=w236:waveform(dbl)[])
        n138 = Multiply(x="TC (s)", y=6.283185307179586) -> (x*y=w302:dbl)
        n139 = Reciprocal(x=w302) -> (1/x=w238:dbl)
        "filter fC (Hz)" <- w238
        n140 = call "decimate_waveforms.vi"("decimating factor"="decimating factor 2", "averaging"=TRUE, "Input Signal"=w236) -> ("Decimated Waveforms"=w235:waveform(dbl)[])  [unwired: 7 in, 1 out]
        n141 = Divide(x=w244, y="decimating factor 2") -> (x/y=w254:dbl)
        n142 = call "Waveform N channels LP pt by pt.vi"("order"="order", "fl"=w238, "fs"=w254, "Array in"=w235) -> ()  [unwired: 7 in, 1 out]
        n143 = for {
          tunnel: [w330] -> w241 mode=indexing
          workers-P: _ -> [_]
          tunnel: w235 -> [w328] mode=indexing
          n144 = Unbundle By Name(w328) -> ("dt"=→"dt":dbl, "Y"=w331:dbl[])
          n145 = call-poly <vilib>:"Mean.vi"("X"=w331) -> ("mean"=w330:dbl)  [unwired: 1 out]
        }
        n146 = Array Size(array=w241) -> (size(s)=w242:i32)
        n147 = Divide(x=w242, y=2) -> (x/y=w240:dbl)
        n148 = Split 1D Array(array=w241, index=w240) -> (first subarray=w305:dbl[], second subarray=w304:dbl[])
        n149 = for {
          tunnel: w305 -> [w386] mode=indexing
          tunnel: w304 -> [w388] mode=indexing
          tunnel: [w387] -> w293 mode=indexing
          n150 = Re/Im To Polar(2:w388, 3:w386) -> (0:w385:dbl, 1:w389:dbl)
          n151 = expression code="x * 180/pi"(w385) -> (w384:dbl)
          n152 = Build Array(w386, w388, w389, w384) -> (w387:dbl[])
        }
        "Results (X, Y, R, Theta)" <- w293
        n153 = call-poly <vilib>:"Basic Averaged DC-RMS.vi"("averaging type"=enum16{"Linear", "Exponential"}."Exponential") -> ()  [unwired: 7 in, 4 out]
        n154 = local read "AO"() -> (w269:T6)
        n155 = Unbundle By Name(w269) -> ("AO amp (V)"=w268:dbl[])
        n156 = global read "Lock-in Globles Multiple Inputs and Outputs used with FGV.vi" "Reset Lockin"() -> (w309:bool)
        n157 = global read "Lock-in Globles Multiple Inputs and Outputs used with FGV.vi" "Stop Lockin"() -> (w315:bool)
        n158 = Transpose 2D Array(2D array=w293) -> (transposed array=w297:dbl[][])
        n159 = Index Array(array=w297) -> (element #1=w300:dbl[], element #2=w299:dbl[], element #3=w298:dbl[], element #4=w279:dbl[])  [unwired: 8 in]
        n160 = Decrement(x="Input Signals") -> (x-1=w277:i16)
        n161 = Array Max & Min(array=w268) -> (max value=w267:dbl)  [unwired: 3 out]
        n162 = case shown="\"X and Y\", Default" "Display" {
          tunnel: w300 -> [w374 _]
          tunnel: [w374 w383] -> w273
          tunnel: w299 -> [w375 _]
          tunnel: [w375 w382] -> w274
          tunnel: w298 -> [_ w383]
          tunnel: w279 -> [_ w382]
          tunnel: [u8 8 ("Display Format:Format") u8 0 ("Display Format:Format")] -> w271
          tunnel: [u8 8 ("Display Format:Format") u8 8 ("Display Format:Format")] -> w270
          tunnel: w267 -> [w371 w379]
          tunnel: [w371 w379] -> w266
          tunnel: [w371 180.0] -> w265
          tunnel: [w370 0.0] -> w264
          tunnel: [w370 -180.0] -> w263
          frame "X and Y", Default {
            n163 = Negate(x=w371) -> (-x=w370:dbl)
          }
          frame "R and Theta" {
          }
        }
        n164 = Or(x=w315, y="stop") -> (x .or. y?=w313:bool)
        n165 = Select(t=4.0 ("f"), s=w313, f=2.0) -> (s? t:f=w312:dbl)
        n166 = Index Array(array=w273, index=w277) -> (element=→"Display 1":dbl)
        n167 = Index Array(array=w274, index=w277) -> (element=→"Display 2":dbl)
        n168 = Get Date/Time In Seconds() -> (seconds since 1Jan1904=w284:timestamp)
        n169 = for {
          tunnel: w273 -> [w367] mode=indexing
          tunnel: w274 -> [w366] mode=indexing
          tunnel: [w365] -> w286 mode=indexing
          tunnel: [w364] -> w285 mode=indexing
          tunnel: w284 -> [w361]
          n170 = Build Array(w366) -> (w362:dbl[])
          n171 = Build Array(w367) -> (w363:dbl[])
          n172 = Bundle By Name("Y"=w363, "t0"=w361) -> (w365:waveform(dbl))  [unwired: 1 in]
          n173 = Bundle By Name("Y"=w362, "t0"=w361) -> (w364:waveform(dbl))  [unwired: 1 in]
        }
        "Display Y (or Theta)" <- w285
        "Display X (or R)" <- w286
        n174 = Select(t=5.0, s=w309, f=w312) -> (s? t:f=w287:dbl)
        n175 = flat-sequence {
          tunnel: [w369] -> w288
          tunnel: w287 -> [w369]
          frame #0 {
            n176 = Wait (ms)(milliseconds to wait="milliseconds to wait") -> ()  [unwired: 1 out]
          }
        }
        n177 = property on="Display 2" class="DigNum (strict)"("Format"=w271) -> ()  [unwired: 2 in, 2 out]
        n178 = property on="Display 1" class="DigNum (strict)"("Format"=w270) -> ()  [unwired: 2 in, 2 out]
        n179 = property on="Display X (or R)" class="WFChart (strict)"("YScale.Maximum"=w266, "YScale.Minimum"=w264) -> ()  [unwired: 2 in, 2 out]
        n180 = property on="Display Y (or Theta)" class="WFChart (strict)"("YScale.Maximum"=w265, "YScale.Minimum"=w263) -> ()  [unwired: 2 in, 2 out]
        n181 = call "Results FGV.vi"("Function"=enum16{"write", "read"}."write", "Input Signals"=w293) -> ()  [unwired: 4 in, 2 out]
      }
      frame 4 {
        # "This code stops the AI/AO Tasks, erases them, and ends program execution."
        n182 = local read "simulate?"() -> (w390:bool)
        n183 = case shown="False" w390 {
          frame False {
            n184 = disable-structure shown="Default" {
              frame condition #0 {
                n185 = local read "AO Task"() -> (w396:refnum<k21>[])
                n186 = local read "AI task"() -> (w397:refnum<k21>[])
                n187 = flat-sequence {
                  tunnel: w397 -> [w410]
                  tunnel: [w409] -> w400
                  tunnel: w396 -> [w409]
                  tunnel: [w408] -> w399
                  tunnel: w400 -> [w416]
                  tunnel: w399 -> [w415]
                  tunnel: [w415] -> w395
                  tunnel: [w414] -> w394
                  frame #0 {
                    n188 = for {
                      tunnel: w410 -> [w413] mode=indexing
                      tunnel: [w411] -> w408 mode=indexing
                      n189 = Wait (ms)(milliseconds to wait=u32 50) -> ()  [unwired: 1 out]
                      n190 = call <vilib>:"DAQmx Stop Task.vi"("task/channels in"=w413) -> ("task out"=w411:refnum<k21>)  [unwired: 13 in, 1 out]
                    }
                  }
                  frame #1 {
                    n191 = for {
                      tunnel: w416 -> [w419] mode=indexing
                      tunnel: [w417] -> w414 mode=indexing
                      n192 = Wait (ms)(milliseconds to wait=u32 50) -> ()  [unwired: 1 out]
                      n193 = call <vilib>:"DAQmx Stop Task.vi"("task/channels in"=w419) -> ("task out"=w417:refnum<k21>)  [unwired: 13 in, 1 out]
                    }
                  }
                }
                n194 = flat-sequence {
                  tunnel: w395 -> [w402]
                  tunnel: w394 -> [w401]
                  tunnel: [w401] -> w398
                  tunnel: w398 -> [w405]
                  frame #0 {
                    n195 = for {
                      tunnel: w402 -> [w404] mode=indexing
                      n196 = call <vilib>:"DAQmx Clear Task.vi"("task in"=w404) -> ()  [unwired: 14 in, 1 out]
                      n197 = Wait (ms)(milliseconds to wait=u32 50) -> ()  [unwired: 1 out]
                    }
                  }
                  frame #1 {
                    n198 = for {
                      tunnel: w405 -> [w407] mode=indexing
                      n199 = call <vilib>:"DAQmx Clear Task.vi"("task in"=w407) -> ()  [unwired: 14 in, 1 out]
                      n200 = Wait (ms)(milliseconds to wait=u32 50) -> ()  [unwired: 1 out]
                    }
                  }
                }
              }
              frame condition #1 (active) {
              }
            }
          }
          frame True {
          }
        }
      }
      frame 5 {
        # "This code stops AI/AO tasks, deletes them, and restarts program execution."
        n201 = local read "simulate?"() -> (w420:bool)
        n202 = case shown="False" w420 {
          frame False {
            n203 = disable-structure shown="TARGET_TYPE==Mac" {
              frame condition #0 {
                n204 = local read "AO Task"() -> (w424:refnum<k21>[])
                n205 = local read "AI task"() -> (w425:refnum<k21>[])
                n206 = flat-sequence {
                  tunnel: w425 -> [w433]
                  tunnel: [w432] -> w430
                  tunnel: w424 -> [w432]
                  tunnel: [w431] -> w429
                  tunnel: w430 -> [w439]
                  tunnel: w429 -> [w438]
                  tunnel: [w438] -> w428
                  tunnel: [w437] -> w427
                  tunnel: w428 -> [w443]
                  tunnel: w427 -> [w444]
                  tunnel: [w444] -> w426
                  tunnel: w426 -> [w447]
                  frame #0 {
                    n207 = for {
                      tunnel: w433 -> [w436] mode=indexing
                      tunnel: [w434] -> w431 mode=indexing
                      n208 = Wait (ms)(milliseconds to wait=u32 50) -> ()  [unwired: 1 out]
                      n209 = call <vilib>:"DAQmx Stop Task.vi"("task/channels in"=w436) -> ("task out"=w434:refnum<k21>)  [unwired: 13 in, 1 out]
                    }
                  }
                  frame #1 {
                    n210 = for {
                      tunnel: w439 -> [w442] mode=indexing
                      tunnel: [w440] -> w437 mode=indexing
                      n211 = Wait (ms)(milliseconds to wait=u32 50) -> ()  [unwired: 1 out]
                      n212 = call <vilib>:"DAQmx Stop Task.vi"("task/channels in"=w442) -> ("task out"=w440:refnum<k21>)  [unwired: 13 in, 1 out]
                    }
                  }
                  frame #2 {
                    n213 = for {
                      tunnel: w443 -> [w446] mode=indexing
                      n214 = call <vilib>:"DAQmx Clear Task.vi"("task in"=w446) -> ()  [unwired: 14 in, 1 out]
                      n215 = Wait (ms)(milliseconds to wait=u32 50) -> ()  [unwired: 1 out]
                    }
                  }
                  frame #3 {
                    n216 = for {
                      tunnel: w447 -> [w449] mode=indexing
                      n217 = call <vilib>:"DAQmx Clear Task.vi"("task in"=w449) -> ()  [unwired: 14 in, 1 out]
                      n218 = Wait (ms)(milliseconds to wait=u32 50) -> ()  [unwired: 1 out]
                    }
                  }
                }
              }
              frame condition #1 (active) {
              }
            }
          }
          frame True {
          }
        }
      }
    }
  }
